vi "Checksum.vi"(1 "input array":u8[](array[numeric]) format="%x") -> (0 "output array":u8[](array[numeric]) format="%x")   [LabVIEW 2014]
panel:
  out "Numeric":u16
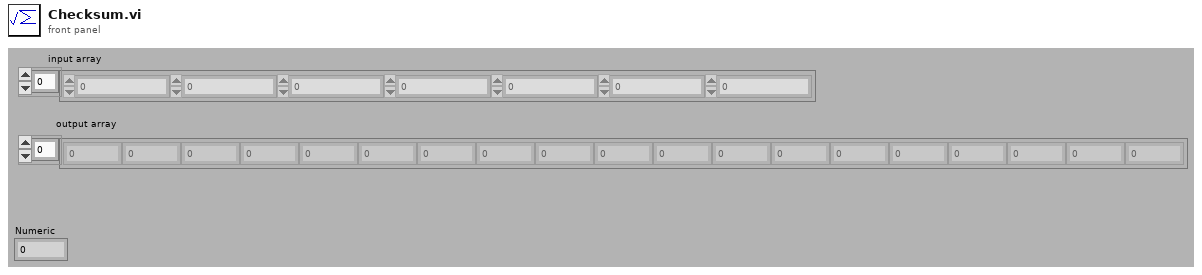
[diagram p1: front panel]
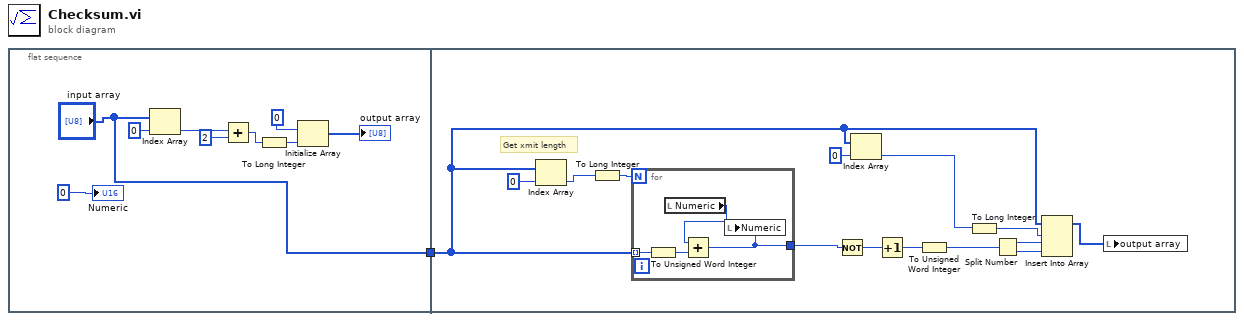
[diagram p0: block diagram]
diagram:
  n1 = flat-sequence {
    tunnel: ["input array"] -> w1
    tunnel: w1 -> [w14]
    frame #0 {
      n2 = Index Array(array="input array", index=0) -> (element=w8:u8)
      n3 = Add(x=w8, y=u8 2) -> (x+y=w4:u8)
      n4 = To Long Integer(number=w4) -> (32bit integer=w3:i32)
      n5 = Initialize Array(u8 0 ("element"), w3) -> (→"output array":u8[])
      "Numeric" <- u16 0 ("Numeric")
    }
    frame #1 {
      # "Get xmit length"
      n6 = Index Array(array=w14, index=0) -> (element=w17:u8)
      n7 = To Long Integer(number=w17) -> (32bit integer=w16:i32)
      n8 = for {
        N: w16 -> [_]
        tunnel: w14 -> [w26] mode=indexing
        tunnel: [w25] -> w13
        n9 = To Unsigned Word Integer(number=w26) -> (unsigned 16bit integer=w28:u16)
        n10 = local read "Numeric"() -> (w27:u16)
        n11 = Add(x=w27, y=w28) -> (x+y=w25:u16)
        n12 = local write "Numeric"(w25) -> ()
      }
      n13 = Not(x=w13) -> (.not. x?=w19:u16)
      n14 = Index Array(array=w14, index=0) -> (element=w12:u8)
      n15 = Increment(x=w19) -> (x+1=w21:u16)
      n16 = To Unsigned Word Integer(number=w21) -> (unsigned 16bit integer=w22:u16)
      n17 = To Long Integer(number=w12) -> (32bit integer=w11:i32)
      n18 = Split Number(x=w22) -> (hi(x)=w23:u8, lo(x)=w24:u8)
      n19 = Insert Into Array(array=w14, index=w11, new element #1=w23, new element #2=w24) -> (w18:u8[])
      n20 = local write "output array"(w18) -> ()
    }
  }
